vi "Set Series View Value.vi"(8 "error in":errorcluster, 9 "Image #":u32, 10 "Image Series":variant[](array[variant]), 11 "Series Graph in":refnum<class "Graph with Series View.lvclass">) -> (0 "error out":errorcluster, 3 "Series Graph out":refnum<class "Graph with Series View.lvclass">)   [LabVIEW 2025, in "Graph with Series View.lvclass"]
uses:
  Graph with Series View.lvclass
  Base Graph/Base Graph.lvclass/Base Graph.ctl
  Graph with Series View.lvclass/Graph with Series View.ctl
  Base Graph/Base Graph.lvclass
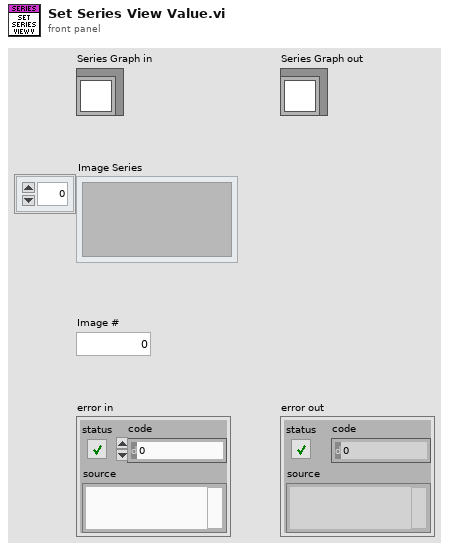
[diagram p1: front panel]
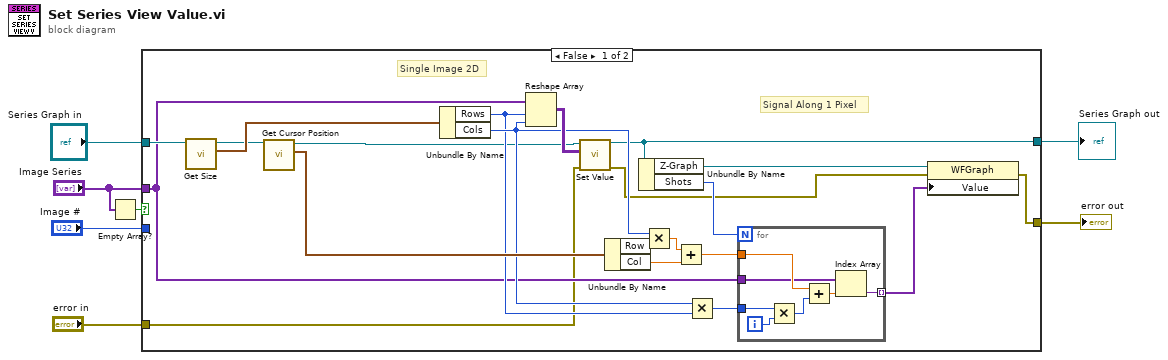
[diagram p0: block diagram]
diagram:
  n1 = Empty Array?(array="Image Series") -> (empty?=w3:bool)
  n2 = case shown="False" w3 {
    tunnel: [w15 w37] -> w7
    tunnel: "Series Graph in" -> [w19 w37]
    tunnel: "Image #" -> [_ _]
    tunnel: "Image Series" -> [w13 _]
    tunnel: "error in" -> [w10 w36]
    tunnel: [w8 w36] -> w1
    frame False {
      # "Signal Along 1 Pixel"
      # "Single Image 2D"
      n3 = call "Get Size.vi"("Base Graph in"=w19) -> ("Size"=w18:cluster{"Rows":u32, "Cols":u32}, "Base Graph out"=w12:refnum<class "Graph with Series View.lvclass">)  [unwired: 9 in]
      n4 = call "Get Cursor Position.vi"("Base Graph in"=w12) -> ("Cursor Position"=w21:cluster{"Col":dbl, "Row":dbl}, "Base Graph out"=w11:refnum<class "Graph with Series View.lvclass">)  [unwired: 9 in]
      n5 = Unbundle By Name(w18) -> ("Rows"=w16:u32, "Cols"=w17:u32)
      n6 = Reshape Array(w13, w16, w17) -> (w20:variant[][])
      n7 = call-dynamic "Set Value.vi"("error in"=w10, "Image"=w20, "Selection Views in"=w11) -> ("error out"=w9:errorcluster, "Selection Views out"=w15:refnum<class "Graph with Series View.lvclass">)  [unwired: 7 in]
      n8 = Unbundle By Name(w21) -> ("Row"=w26:dbl, "Col"=w27:dbl)
      n9 = Unbundle By Name(w15) -> ("Z-Graph"=w23:refnum<vi>, "Shots"=w24:u32)
      n10 = Multiply(x=w17, y=w26) -> (x*y=w25:dbl)
      n11 = Add(x=w25, y=w27) -> (x+y=w14:dbl)
      n12 = Multiply(x=w17, y=w16) -> (x*y=w22:u32)
      n13 = for {
        N: w24 -> [_]
        tunnel: w13 -> [w30]
        tunnel: w22 -> [w34]
        tunnel: w14 -> [w31]
        tunnel: [w29] -> w28 mode=indexing
        i -> [w35]
        n14 = Multiply(x=w34, y=w35) -> (x*y=w32:u32)
        n15 = Add(x=w31, y=w32) -> (x+y=w33:dbl)
        n16 = Index Array(array=w30, index=w33) -> (element=w29:variant)
      }
      n17 = property class="WFGraph"(reference=w23, error in=w9, "Value"=w28) -> (error out=w8:errorcluster)  [unwired: 1 out]
    }
    frame True {
    }
  }
  "Series Graph out" <- w7
  "error out" <- w1
